vi "get_FP_BD_images.vi"(8 "error in (no error)":errorcluster, 11 "VI Path":path) -> (0 "error out":errorcluster, 1 "VI Ref":refnum<vi>, 2 "VI Name":string, 3 "Control details":string, 4 "Control Labels":string[](array[string]), 5 "Images Folder":path, 6 "Control References":refnum<vi>[](array[refnum]), 7 "Indicator/Control":bool[](array[boolean]))   [LabVIEW 2020, in "lv_documentation.lvlib"]
uses:
  lv_documentation.lvlib
  <vilib>/Utility/traverseref.llb/TRef TravTarget.ctl
  <vilib>/Utility/sysdir.llb/System Directory Type.ctl
  <vilib>/Utility/traverseref.llb/VI Scripting - Traverse.lvlib
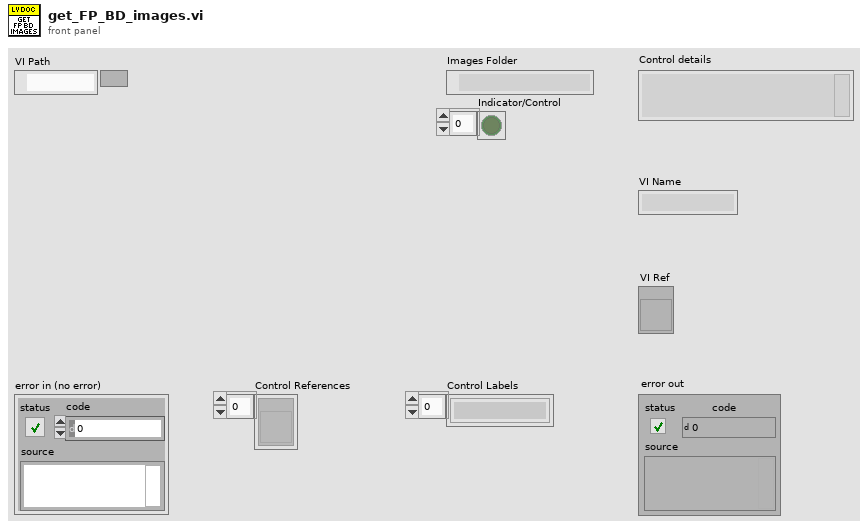
[diagram p1: front panel]
types:
  T1 = typedef "System Directory Type.ctl" = i32
  T2 = typedef "TRef TravTarget.ctl" = enum16{"FP", "BD", "Other"}
  T3 = typedef "imagedata.ctl" = cluster{"image type":i32, "image depth":i32, "image":u8[], "mask":u8[], "colors":u32[], "Rectangle":cluster{"left":i16, "top":i16, "right":i16, "bottom":i16}}
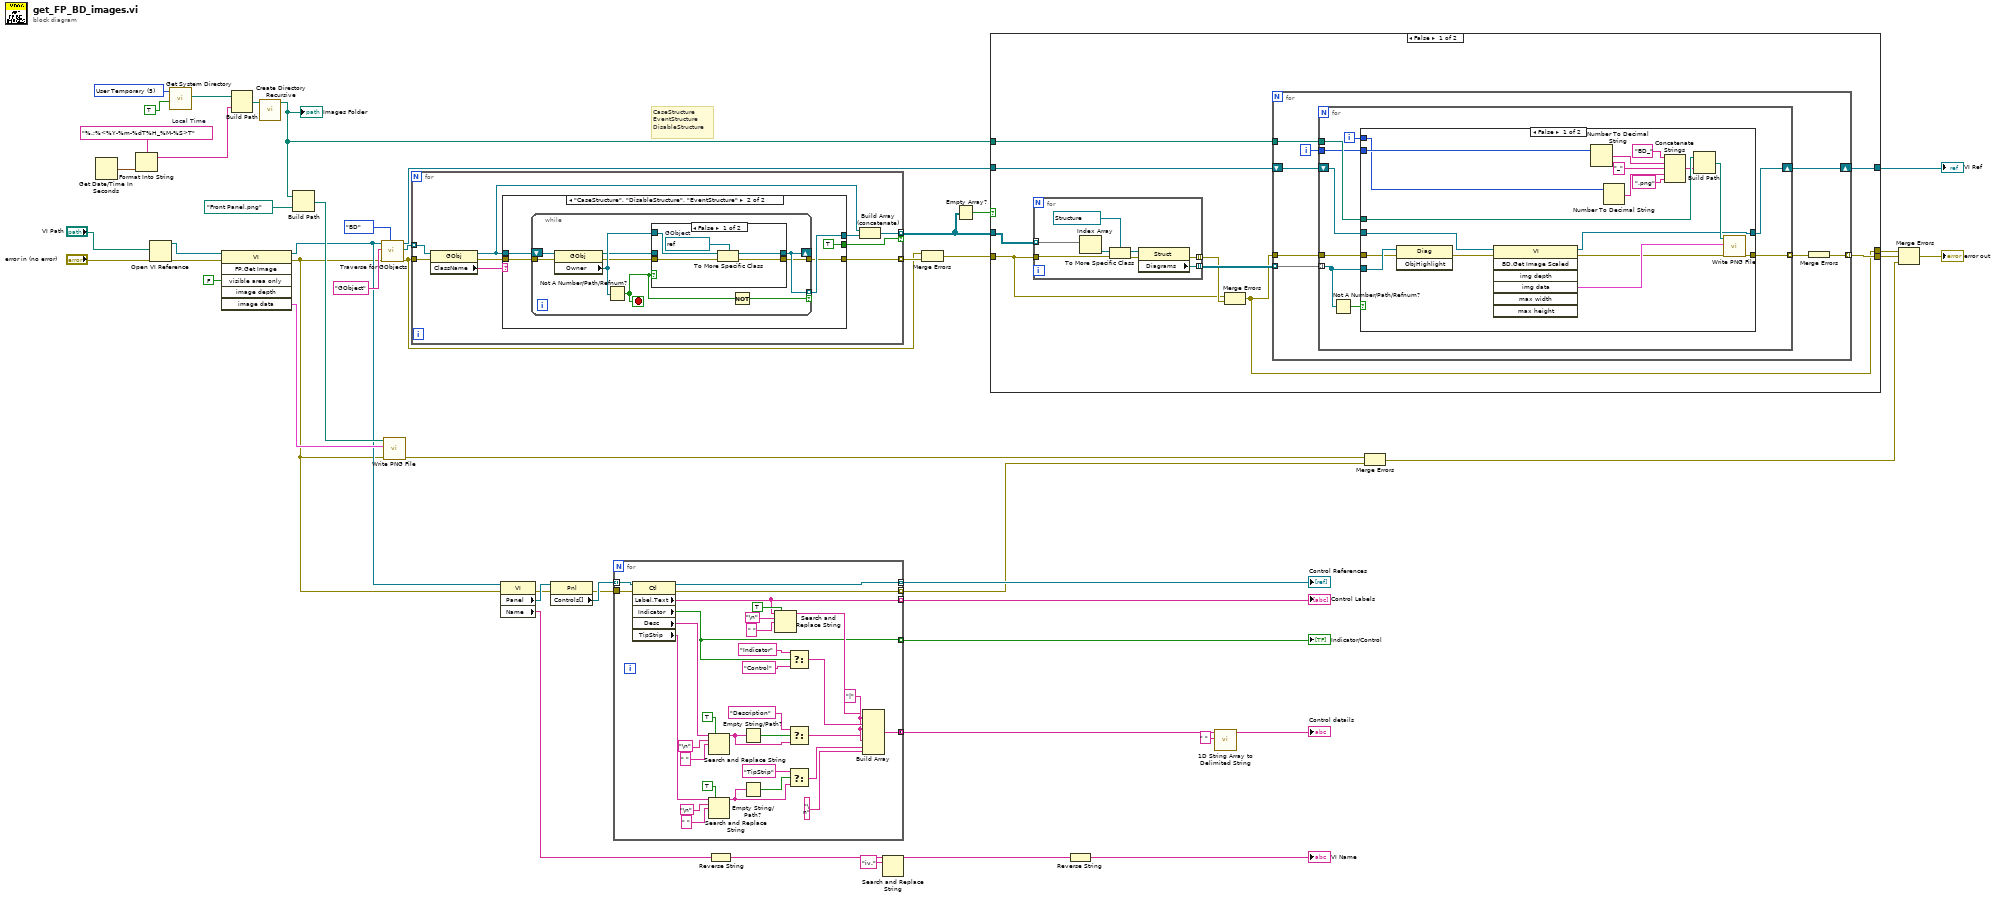
[diagram p0: block diagram]
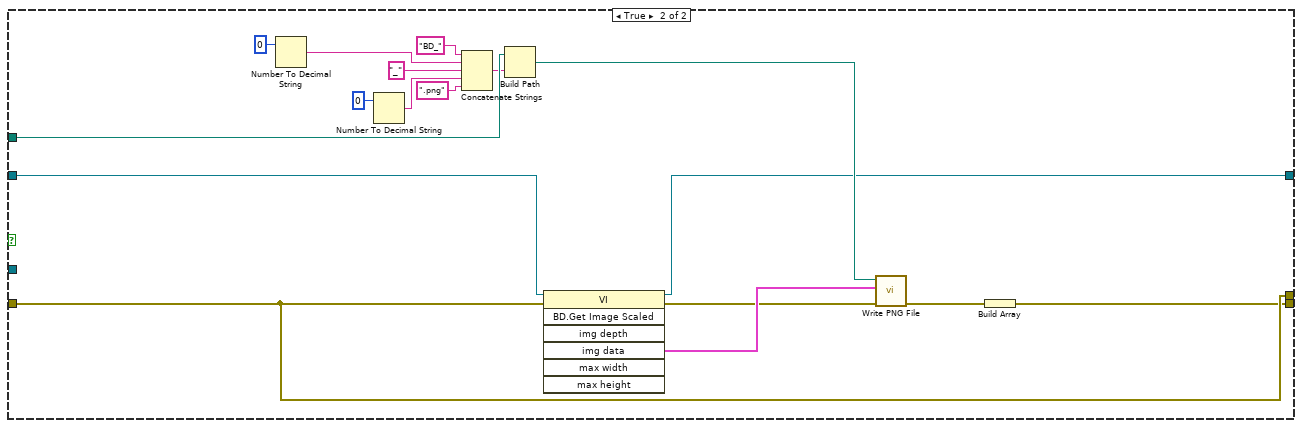
[diagram p3: hidden frame]
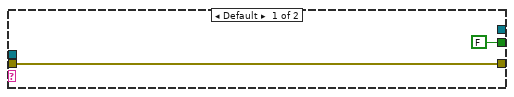
[diagram p4: hidden frame]
diagram:
  w10 = "%.;%<%Y-%m-%dT%H_%M-%S>T"  # Local Time
  w13 = T1 5 items=["User Home"=0, "User Desktop"=1, "User Documents"=2, "User Application Data"=3, "User Preferences"=4, "User Temporary"=5, "Public Documents"=6, "Public Application Data"=7, "Public Preferences"=8, "Public Cache"=13, "System Core Libraries"=9, "System Installed Libraries"=10, "Application Files"=11, "Boot Volume Root"=12] ("system directory type")
  # "CaseStructure\nEventStructure\nDisableStructure"
  n1 = Get Date/Time In Seconds() -> (seconds since 1Jan1904=w9:timestamp)
  n2 = Format Into String(format string=w10, w9) -> (resulting string=w8:string)  [unwired: 2 in, 1 out]
  n3 = Open VI Reference(vi path="VI Path", error in (no error)="error in (no error)") -> (vi reference=w39:refnum<vi>, error out=w37:errorcluster)  [unwired: 4 in]
  n4 = call <vilib>:"Get System Directory.vi"("create directory if not found? (F)"=TRUE, "system directory type"=w13) -> ("system directory"=w11:path)  [unwired: 9 in]
  n5 = invoke class="VI" method="FP.Get Image"(reference=w39, error in=w37, "visible area only"=FALSE ("Visible Area Only")) -> (reference out=w27:refnum<vi>, error out=w6:errorcluster, "image data"=w49:T3)  [unwired: 3 in, 3 out]
  n6 = Build Path(base path=w11, name or relative path=w8) -> (appended path=w7:path)
  n7 = call <vilib>:"Create Directory Recursive.vi"("directory"=w7) -> ("directory copy"=w41:path)  [unwired: 4 in, 2 out]
  "Images Folder" <- w41
  n8 = Build Path(base path=w41, name or relative path=path "Front Panel.png") -> (appended path=w46:path)
  n9 = call <vilib>:"Traverse for GObjects.vi"("Traverse Target"=TRef_TravTarget."BD", "error in (no error)"=w6, "Class Name"="GObject", "VI Refnum"=w27) -> ("error out"=w35:errorcluster, "References"=w44:refnum<vi>[], "dup VI Refnum"=w42:refnum<vi>)  [unwired: 4 in, 1 out]
  n10 = call <vilib>:"Write PNG File.vi"("error in (no error)"=w6, "image data"=w49, "path to PNG file"=w46) -> ("error out"=w31:errorcluster)  [unwired: 7 in, 1 out]
  n11 = for {
    tunnel: w44 -> [w58] mode=indexing
    tunnel: [w54] -> w29 mode=indexing if=w53
    tunnel: w35 -> [w52]
    tunnel: [w50] -> w36 mode=indexing
    n12 = property class="GObj"(reference=w58, error in=w52) -> (reference out=w55:refnum<vi>, error out=w51:errorcluster, "ClassName"=w57:string)
    n13 = case shown="\"CaseStructure\", \"DisableStructure\", \"EventStructure\"" w57 {
      tunnel: [FALSE TRUE] -> w53
      tunnel: w55 -> [_ w64]
      tunnel: [_ w63] -> w56
      tunnel: w51 -> [w59 w62]
      tunnel: [w59 w61] -> w50
      frame Default {
      }
      frame "CaseStructure", "DisableStructure", "EventStructure" {
        n14 = while {
          shift-right: [w71] -> _
          shift-left: w64 -> [w74]
          tunnel: [w71] -> w63 mode=indexing if=w69
          tunnel: w62 -> [w68]
          tunnel: [w66] -> w61
          stop <- w70 stop-if-true
          n15 = property class="GObj"(reference=w74, error in=w68) -> (reference out=w72:refnum<vi>, error out=w67:errorcluster, "Owner"=w73:refnum<vi>)
          n16 = Not A Number/Path/Refnum?(number/path/refnum=w73) -> (NaN/Path/Refnum?=w70:bool)
          n17 = case shown="False" w70 {
            tunnel: w73 -> [w78 _]
            tunnel: [w77 w81] -> w71
            tunnel: w72 -> [_ w81]
            tunnel: w67 -> [w76 w80]
            tunnel: [w75 w80] -> w66
            frame False {
              w79 = refnum<vi> refnum  # GObject
              n18 = To More Specific Class(target class=w79, reference=w78, error in=w76) -> (specific class reference=w77:refnum<vi>, error out=w75:errorcluster)
            }
            frame True {
            }
          }
          n19 = Not(x=w70) -> (.not. x?=w69:bool)
        }
      }
    }
    n20 = Build Array (concatenate)(w55, w56) -> (w54:refnum<vi>[])
  }
  n21 = property class="VI"(reference=w27, error in=w6) -> (error out=w5:errorcluster, "Panel"=w26:refnum<vi>, "Name"=w22:string)  [unwired: 1 out]
  n22 = property class="Pnl"(reference=w26, error in=w5) -> (error out=w4:errorcluster, "Controls[]"=w25:refnum<vi>[])  [unwired: 1 out]
  n23 = for {
    tunnel: w25 -> [w113] mode=indexing
    tunnel: [w109] -> w14 mode=concatenating
    tunnel: [w101] -> w16 mode=indexing
    tunnel: [w100] -> w15 mode=indexing
    tunnel: w4 -> [w91]
    tunnel: [w90] -> w2 mode=indexing
    tunnel: [w82] -> w1 mode=indexing
    w108 = "|" ("element")
    n24 = property class="Ctl"(reference=w113, error in=w91) -> (reference out=w101:refnum<vi>, error out=w90:errorcluster, "Label.Text"=w100:string, "Indicator"=w82:bool, "Desc"=w106:string, "TipStrip"=w105:string)
    n25 = Search and Replace String(replace all?=TRUE ("replace all? (F)"), input string=w106, search string="\n", replace string=" " ("replace string (\"\")")) -> (result string=w93:string)  [unwired: 4 in, 3 out]
    n26 = Search and Replace String(replace all?=TRUE ("replace all? (F)"), input string=w105, search string="\n", replace string=" " ("replace string (\"\")")) -> (result string=w95:string)  [unwired: 4 in, 3 out]
    n27 = Empty String/Path?(string/path=w93) -> (empty?=w99:bool)
    n28 = Empty String/Path?(string/path=w95) -> (empty?=w96:bool)
    n29 = Search and Replace String(replace all?=TRUE ("replace all? (F)"), input string=w100, search string="\n", replace string=" " ("replace string (\"\")")) -> (result string=w107:string)  [unwired: 4 in, 3 out]
    n30 = Select(t="Indicator" ("Label.Text"), s=w82, f="Control" ("Label.Text")) -> (s? t:f=w110:string)
    n31 = Select(t="Description", s=w99, f=w93) -> (s? t:f=w92:string)
    n32 = Select(t="TipStrip", s=w96, f=w95) -> (s? t:f=w94:string)
    n33 = Build Array(w107, w108, w110, w108, w92, w108, w94, "\n" ("element")) -> (w109:string[])
  }
  "Control References" <- w16
  "Control Labels" <- w15
  "Indicator/Control" <- w1
  n34 = Reverse String(1:w22) -> (0:w20:string)
  n35 = Search and Replace String(input string=w20, search string="iv.") -> (result string=w21:string)  [unwired: 6 in, 3 out]
  n36 = Merge Errors(w35, w36) -> (w34:errorcluster)
  n37 = Empty Array?(array=w29) -> (empty?=w28:bool)
  n38 = case shown="False" w28 {
    tunnel: w29 -> [w122 _]
    tunnel: w42 -> [w120 w184]
    tunnel: w41 -> [w119 w183]
    tunnel: w34 -> [w117 w182]
    tunnel: [w116 w169] -> w33
    tunnel: [w115 w182] -> w32
    tunnel: [w114 w168] -> w17
    frame False {
      n39 = for {
        tunnel: w122 -> [w167] mode=indexing
        tunnel: [w163] -> w121 mode=indexing
        tunnel: w117 -> [w162]
        tunnel: [w160] -> w118 mode=indexing
        n40 = Index Array(array=w167) -> (element=w166:refnum<vi>)  [unwired: 1 in]
        n41 = To More Specific Class(target class=refnum<vi> refnum ("specific class reference"), reference=w166, error in=w162) -> (specific class reference=w165:refnum<vi>, error out=w161:errorcluster)
        n42 = property class="Struct"(reference=w165, error in=w161) -> (error out=w160:errorcluster, "Diagrams"=w163:refnum<vi>[])  [unwired: 1 out]
      }
      n43 = Merge Errors(w117, w118) -> (w115:errorcluster)
      n44 = for {
        tunnel: w121 -> [w130] mode=indexing
        tunnel: w119 -> [w128]
        tunnel: w115 -> [w126]
        tunnel: [w124] -> w116 mode=indexing
        shift-right: [w123] -> w114
        shift-left: w120 -> [w129]
        i -> [w127]
        n45 = for {
          tunnel: w130 -> [w133] mode=indexing
          tunnel: w128 -> [w138]
          tunnel: w127 -> [w137]
          tunnel: w126 -> [w135]
          tunnel: [w134] -> w125 mode=indexing
          shift-right: [w131] -> w123
          shift-left: w129 -> [w139]
          i -> [w136]
          n46 = Not A Number/Path/Refnum?(number/path/refnum=w133) -> (NaN/Path/Refnum?=w132:bool)
          n47 = case shown="False" w132 {
            tunnel: w133 -> [w157 _]
            tunnel: w139 -> [w156 w158]
            tunnel: w138 -> [w154 _]
            tunnel: w137 -> [w150 _]
            tunnel: w136 -> [w149 _]
            tunnel: w135 -> [w144 w159]
            tunnel: [w141 w159] -> w134
            tunnel: [w140 w158] -> w131
            frame False {
              n48 = invoke class="Diag" method="ObjHighlight"(reference=w157, error in=w144) -> (error out=w143:errorcluster)  [unwired: 1 in, 2 out]
              n49 = invoke class="VI" method="BD.Get Image Scaled"(reference=w156, error in=w143) -> (reference out=w140:refnum<vi>, error out=w142:errorcluster, "img data"=w155:T3)  [unwired: 5 in, 4 out]
              n50 = Number To Decimal String(number=w150) -> (decimal integer string=w148:string)  [unwired: 1 in]
              n51 = Number To Decimal String(number=w149) -> (decimal integer string=w147:string)  [unwired: 1 in]
              n52 = Concatenate Strings("BD_" ("string"), w148, "_" ("string"), w147, ".png" ("string")) -> (w153:string)
              n53 = Build Path(base path=w154, name or relative path=w153) -> (appended path=w145:path)
              n54 = call <vilib>:"Write PNG File.vi"("error in (no error)"=w142, "image data"=w155, "path to PNG file"=w145) -> ("error out"=w141:errorcluster)  [unwired: 7 in, 1 out]
            }
            frame True {
            }
          }
        }
        n55 = Merge Errors(w125) -> (w124:errorcluster)
      }
    }
    frame True {
      n56 = Number To Decimal String(number=0) -> (decimal integer string=w177:string)  [unwired: 1 in]
      n57 = Number To Decimal String(number=0) -> (decimal integer string=w176:string)  [unwired: 1 in]
      n58 = Concatenate Strings("BD_" ("string"), w177, "_" ("string"), w176, ".png" ("string")) -> (w180:string)
      n59 = Build Path(base path=w183, name or relative path=w180) -> (appended path=w174:path)
      n60 = invoke class="VI" method="BD.Get Image Scaled"(reference=w184, error in=w182) -> (reference out=w168:refnum<vi>, error out=w173:errorcluster, "img data"=w181:T3)  [unwired: 5 in, 4 out]
      n61 = call <vilib>:"Write PNG File.vi"("error in (no error)"=w173, "image data"=w181, "path to PNG file"=w174) -> ("error out"=w170:errorcluster)  [unwired: 7 in, 1 out]
      n62 = Build Array(w170) -> (w169:errorcluster[])
    }
  }
  "VI Ref" <- w17
  n63 = Reverse String(1:w21) -> (0:→"VI Name":string)
  n64 = call <vilib>:"1D String Array to Delimited String.vi"("delimiter"=" ", "string array"=w14) -> ("delimited string"=→"Control details":string)  [unwired: 9 in]
  n65 = Merge Errors(w31, w2) -> (w3:errorcluster)
  n66 = Merge Errors(w32, w33, w3) -> (→"error out":errorcluster)
